vi "Steam.vi"(8 "error in (no error)":errorcluster, 11 "Chef in":refnum<class "Chef.lvclass">) -> (0 "error out":errorcluster, 3 "Chef out":refnum<class "Chef.lvclass">)   [LabVIEW 2011, in "Chef.lvclass"]
uses:
  Chef.lvclass
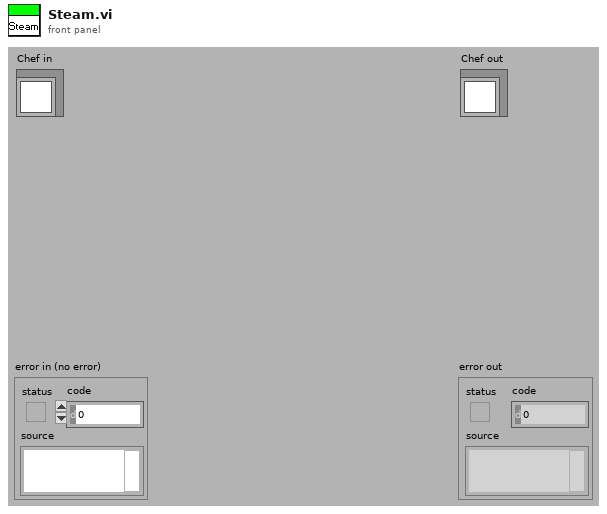
[diagram p1: front panel]
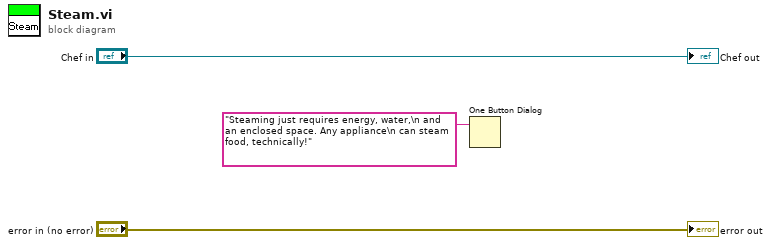
[diagram p0: block diagram]
diagram:
  n1 = One Button Dialog(message="Steaming just requires energy, water,\n and an enclosed space. Any appliance\n can steam food, technically!") -> ()  [unwired: 1 in, 1 out]
  "error out" <- "error in (no error)"
  "Chef out" <- "Chef in"
